vi "CutROI.vi"(0 "Full Image In":dbl[][](graph), 5 "Col Start":dbl, 7 "Col End":dbl, 9 "Row Start":dbl, 11 "Row End":dbl) -> (8 "Cut Image Out":dbl[][](graph))   [LabVIEW 2013]
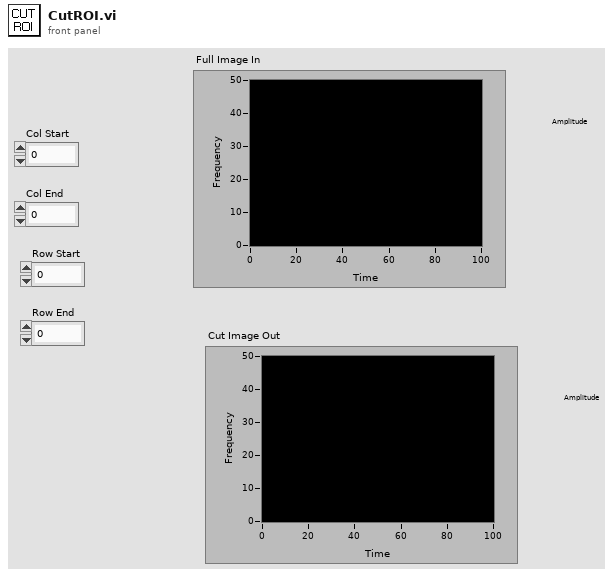
[diagram p1: front panel]
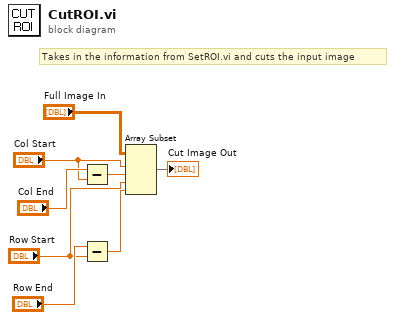
[diagram p0: block diagram]
diagram:
  # "Takes in the information from SetROI.vi and cuts the input image"
  n1 = Subtract(x="Col End", y="Col Start") -> (x-y=w6:dbl)
  n2 = Subtract(x="Row End", y="Row Start") -> (x-y=w3:dbl)
  n3 = Array Subset(array="Full Image In", index (row)="Col Start", length (row)=w6, index (col)="Row Start", length (col)=w3) -> (→"Cut Image Out":dbl[][])
